vi "get_number_of_samples.vi"(8 "error in (no error)":errorcluster, 11 "StimulatorDL090503 in":refnum<class "StimulatorDL090503.lvclass">) -> (0 "error out":errorcluster, 2 "number of samples":i32, 3 "StimulatorDL090503 out":refnum<class "StimulatorDL090503.lvclass">)   [LabVIEW 2010, in "StimulatorDL090503.lvclass"]
uses:
  StimulatorDL090503.lvclass
  StimulatorDL090503.lvclass/StimulatorDL090503.ctl
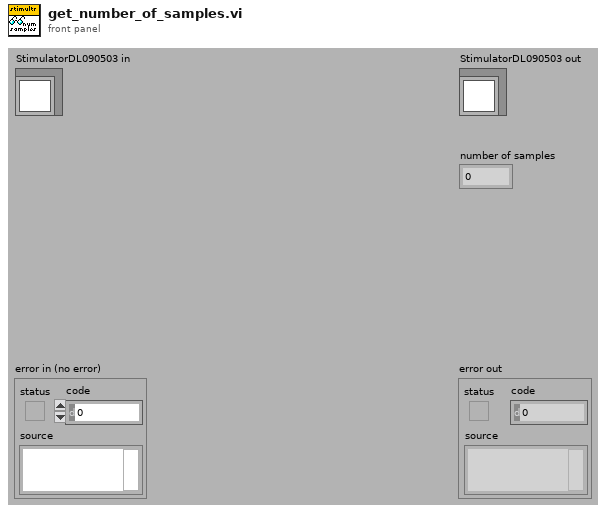
[diagram p1: front panel]
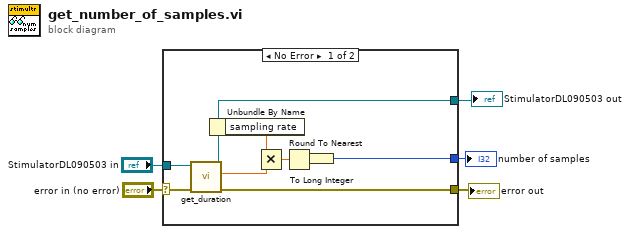
[diagram p0: block diagram]
diagram:
  n1 = case shown="No Error" "error in (no error)" {
    selector: "error in (no error)" -> [w11 w16]
    tunnel: [w10 w16] -> w4
    tunnel: [w7 w15] -> w3
    tunnel: "StimulatorDL090503 in" -> [w8 w15]
    tunnel: [w9 _] -> w5
    frame No Error {
      n2 = call-dynamic "get_duration.vi"("error in (no error)"=w11, "DL090503StimulatorScaffold.lvclass in"=w8) -> ("error out"=w10:errorcluster, "duration"=w12:dbl[unit], "DL090503StimulatorScaffold.lvclass out"=w7:refnum<class "StimulatorDL090503.lvclass">)  [unwired: 7 out]
      n3 = Unbundle By Name(w7) -> ("sampling rate"=w6:dbl[unit])
      n4 = Multiply(x=w6, y=w12) -> (x*y=w13:dbl)
      n5 = Round To Nearest(number=w13) -> (nearest integer value=w14:dbl)
      n6 = To Long Integer(number=w14) -> (32bit integer=w9:i32)
    }
    frame Error {
    }
  }
  "error out" <- w4
  "StimulatorDL090503 out" <- w3
  "number of samples" <- w5
